vi "RemoveCalibration.vi"(2 "Excitations":dbl[](array[numeric]), 3 "# always zero":i32, 5 "Calibrations":T1 {"Offset (V)" format="%_6p"; "Gain" format="%_6p"}) -> (1 "Potentials":dbl[](array[numeric]))   [LabVIEW 2018]
uses:
  Calibrations.ctl
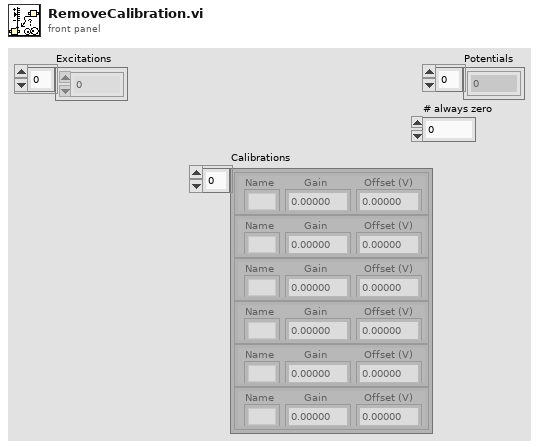
[diagram p1: front panel]
types:
  T1 = typedef "Calibrations.ctl" = cluster{"Gain":dbl, "Offset (V)":dbl, "Name":string}[]
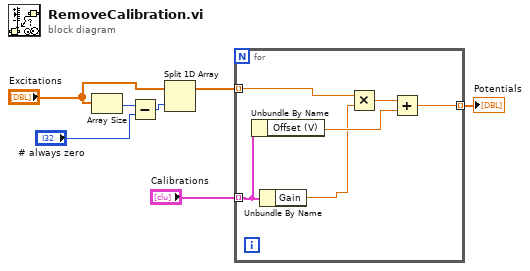
[diagram p0: block diagram]
diagram:
  n1 = Array Size(array="Excitations") -> (size(s)=w5:i32)
  n2 = Subtract(x=w5, y="# always zero") -> (x-y=w3:i32)
  n3 = Split 1D Array(array="Excitations", index=w3) -> (first subarray=w1:dbl[])  [unwired: 1 out]
  n4 = for {
    tunnel: "Calibrations" -> [w13] mode=indexing
    tunnel: w1 -> [w12] mode=indexing
    tunnel: [w9] -> w6 mode=indexing
    n5 = Unbundle By Name(w13) -> ("Offset (V)"=w10:dbl)
    n6 = Unbundle By Name(w13) -> ("Gain"=w8:dbl)
    n7 = Multiply(x=w12, y=w8) -> (x*y=w11:dbl)
    n8 = Add(x=w11, y=w10) -> (x+y=w9:dbl)
  }
  "Potentials" <- w6
